vi "Initialization VI.vi"(8 "error in (no error)":errorcluster, 10 "Custom XML":string, 11 "Device Item Ref in":T1 format="%.0x") -> (0 "error out":errorcluster, 3 "Device Item Ref out":T1 format="%.0x")   [LabVIEW 2019, in "J1939 Addon System Explorer.lvlib"]
uses:
  J1939 Addon System Explorer.lvlib
  <vilib>/NI VeriStand/Custom Device API/Custom Device Item Ref.ctl
  Addon Shared/J1939 Addon Shared.lvlib
  <vilib>/NI VeriStand/Custom Device API/Custom Device API.lvlib
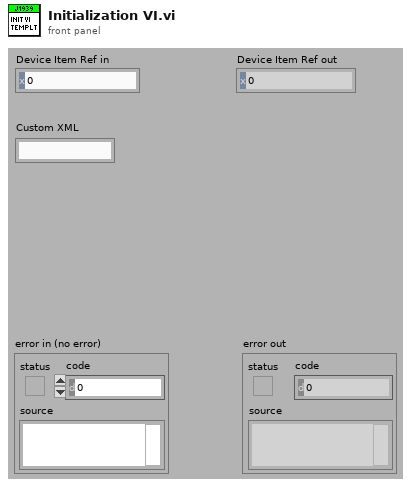
[diagram p1: front panel]
types:
  T1 = typedef "Custom Device API.lvlib/Custom Device Item Ref.ctl" = u64
  T2 = typedef "J1939 Addon Shared.lvlib/Monitor Settings.ctl" = cluster{"Address":u8, "Name":u64, "Include DA":bool}
  T3 = typedef "J1939 Addon Shared.lvlib/XNET Settings.ctl" = cluster{"Database":refnum<k21>, "Cluster":refnum<k21>, "Port":string, "Baud rate [Bd]":u32, "Termination":u32, "Incoming Decimation":u32, "Outgoing Decimation":u32}
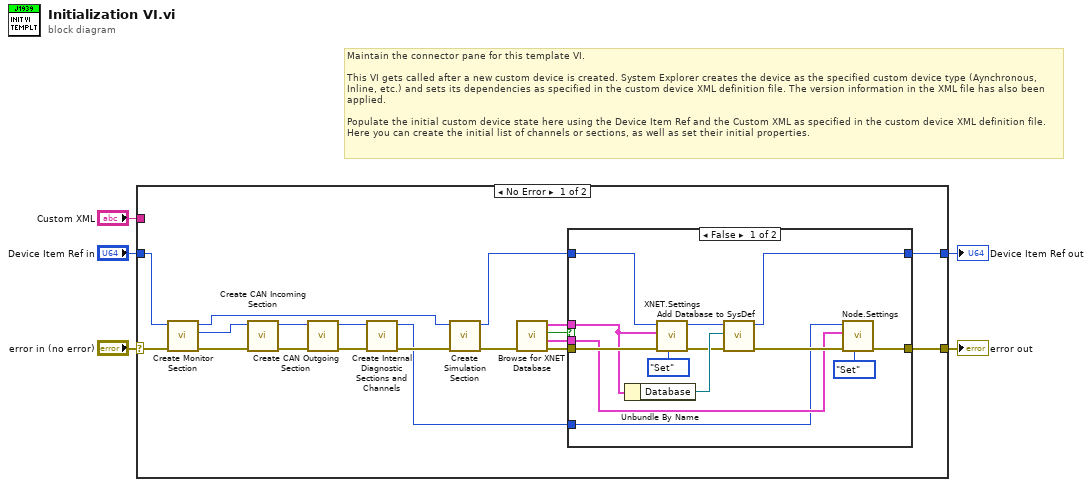
[diagram p0: block diagram]
diagram:
  # "Maintain the connector pane for this template VI.\n\nThis VI gets called after a new custom device is created. System Explorer creates the device as the specified custom device type (Aynchronous, Inline, etc.) and sets its dependencies as specified in the custom device XML definition file. The version information in the XML file has also been applied.\n\nPopulate the initial custom device state here using the Device Item Ref and the Custom XML as specified in the custom device XML definition file. Here you can create the initial list of channels or sections, as well as set their initial properties."
  n1 = case shown="No Error" "error in (no error)" {
    selector: "error in (no error)" -> [w13 w41]
    tunnel: [w22 w41] -> w5
    tunnel: [w18 w40] -> w3
    tunnel: "Device Item Ref in" -> [w11 w40]
    tunnel: "Custom XML" -> [_ _]
    frame No Error {
      n2 = call "Create Monitor Section.vi"("error in (no error)"=w13, "Device Item Ref in"=w11) -> ("error out"=w12:errorcluster, "Section Ptr"=w6:T1, "Parent Ref out"=w7:T1)  [unwired: 7 in]
      n3 = call "Create CAN Incoming Section.vi"("error in (no error)"=w12, "Device Item Ref in"=w6) -> ("error out"=w24:errorcluster, "Device Item Ref Out"=w23:T1)  [unwired: 8 in]
      n4 = call "Create CAN Outgoing Section.vi"("error in (no error)"=w24, "Parent Ref in"=w23) -> ("error out"=w16:errorcluster, "Parent Ref out"=w17:T1)  [unwired: 8 in]
      n5 = call "Create Internal Diagnostic Sections and Channels.vi"("error in (no error)"=w16, "Device Item Ref in"=w17) -> ("error out"=w15:errorcluster, "Device Item Ref Out"=w8:T1)  [unwired: 8 in]
      n6 = call "Create Simulation Section.vi"("error in (no error)"=w15, "Parent Ref in"=w7) -> ("error out"=w14:errorcluster, "Parent Ref out"=w10:T1)  [unwired: 7 in, 1 out]
      n7 = call "Browse for XNET Database.vi"("error in (no error)"=w14) -> ("error out"=w21:errorcluster, "J1939 Monitor Settings"=w9:T2, "Cancel Out"=w20:bool, "J1939 XNET Settings"=w19:T3)  [unwired: 7 in]
      n8 = case shown="False" w20 {
        tunnel: [w25 w39] -> w22
        tunnel: w21 -> [w35 w39]
        tunnel: w19 -> [w34 _]
        tunnel: w10 -> [w32 w38]
        tunnel: [w37 w38] -> w18
        tunnel: w9 -> [w28 _]
        tunnel: w8 -> [w27 _]
        frame False {
          n9 = Unbundle By Name(w34) -> ("Database"=w36:refnum<k21>)
          n10 = call "XNET.Settings.vi"("Action"=enum8{"Get", "Set"}."Set", "error in (no error)"=w35, "J1939 XNET Settings"=w34, "Parent Ref in"=w32) -> ("error out"=w33:errorcluster, "Item Ref out"=w31:T1)  [unwired: 5 in, 1 out]
          n11 = call "Add Database to SysDef.vi"("error in"=w33, "DB Alias"=w36, "Item Ref in"=w31) -> ("error out"=w29:errorcluster, "Item Ref out"=w37:T1)  [unwired: 7 in]
          n12 = call "Node.Settings.vi"("Action"=enum8{"Get", "Set"}."Set", "error in (no error)"=w29, "Node.Settings"=w28, "Item Ref in"=w27) -> ("error out"=w25:errorcluster)  [unwired: 5 in, 2 out]
        }
        frame True {
        }
      }
    }
    frame Error {
    }
  }
  "error out" <- w5
  "Device Item Ref out" <- w3
